vi "unpack_microphone_s16.vi"(10 "payload_size":u32, 11 "payload":u64) -> (2 "error":bool, 3 "samples":i16[](array[numeric]))   [LabVIEW 2023]
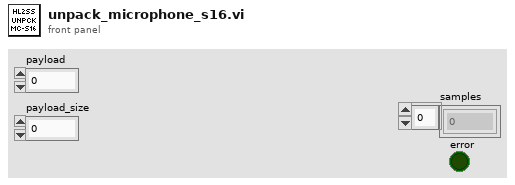
[diagram p1: front panel]
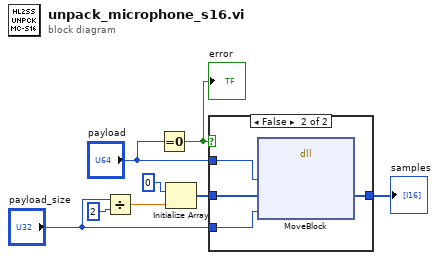
[diagram p0: block diagram]
diagram:
  n1 = Divide(x="payload_size", y=u32 2) -> (x/y=w6:dbl)
  n2 = Equal To 0?(x="payload") -> (x = 0?=w7:bool)
  "error" <- w7
  n3 = Initialize Array(i16 0 ("payload_size"), w6) -> (w5:i16[])
  n4 = case shown="False" w7 {
    tunnel: "payload" -> [_ w12]
    tunnel: "payload_size" -> [_ w13]
    tunnel: w5 -> [w9 w11]
    tunnel: [w9 w10] -> w1
    frame True {
    }
    frame False {
      n5 = dll-call lib="LabVIEW" fn="MoveBlock"("ps"=w12, "pd"=w11, "size"=w13) -> ("pd"=w10:i16[])  [unwired: 6 in, 2 out]
    }
  }
  "samples" <- w1
